vi "Write Enable Bias.vi"(10 "Enable Bias":bool, 11 "LCR-Measurement in":refnum<class "OTP_LCR_Meas.lvclass">) -> (3 "LCR-Measurement out":refnum<class "OTP_LCR_Meas.lvclass">)   [LabVIEW 2020, in "OTP_LCR_Meas.lvclass"]
uses:
  OTP_LCR_Meas.lvclass
  OTP_LCR_Meas.lvclass/OTP_LCR_Meas.ctl
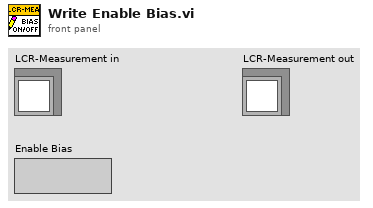
[diagram p1: front panel]
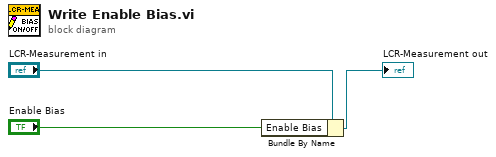
[diagram p0: block diagram]
diagram:
  n1 = Bundle By Name(cluster="LCR-Measurement in", "Enable Bias"="Enable Bias") -> (→"LCR-Measurement out":refnum<class "OTP_LCR_Meas.lvclass">)
